vi "SPI Read Write.vi"(0 "SPI_Port":i8, 1 "SPI_CPOL":bool, 2 "SPI_CPHA":bool, 5 "SPI_Clock Divider":u32=20, 7 "SPI_Total Bytes":u16=1, 9 "SPI_Total Bits":u16=8, 11 "SPI_Write Data":u8[](array[numeric])=[0, 0], 12 "SPI_CS Active State":bool caption="SPI_CS\nActive State", 13 "SPI_CS":u8=1 format="%08b") -> (4 "SPI_Read Data":u8[](array[numeric]))   [LabVIEW 2019]
uses:
  Controls/FPGA SPI_FPGA SPI State.ctl
  <vilib>/rvi/Emulation/niFpgaSctlEmulationGetInTimedLoop.vi
  FPGA SPI_Globals.vi
  <vilib>/rvi/Emulation/niFpgaProcessEmulError.vi
  <vilib>/rvi/Emulation/niFpgaGetClockAttributes.vi
  <vilib>/rvi/Emulation/niFpgaEmulationReportErrorSimple.vi
  <vilib>/rvi/Emulation/niFpgaCriticalErrorInLSC.vi
  <vilib>/rvi/Emulation/niFpgaEmulationIsFPGAContextNoSignature.vi
  <vilib>/rvi/errors/niFpgaSetErrorForExecOnDevCompSimple.vi
  <vilib>/rvi/eio/common/nirviEmuReportErrorAndStop.vi
  <vilib>/rvi/DataTransferAndStorage/Container/Common/niFpgaContainerGetUniqueNameForEmu.vi
  <vilib>/rvi/FIFO/Fifo_Resource/nirvififoEmulationSetSize.vi
  <vilib>/rvi/FIFO/Fifo_Resource/nirviFifoEmulationQueueMgr.vi
  <instcachedir>/0/nirviFifoEmulationQueueMgr_E5CAEC123FF24DC58D834DCA3CDAA9B5.lvgen/nirviFifoEmulationQueueMgr_E5CAEC123FF24DC58D834DCA3CDAA9B5_002.vi
  <vilib>/rvi/FIFO/Fifo_Resource/nirvififoEmulationDetermineInputValidOut.vi
  <vilib>/rvi/FIFO/Fifo_Resource/nirvififoEmulationCreateLock.vi
  <vilib>/rvi/FIFO/Fifo_Resource/nirvififoEmulationObtainLock.vi
  <vilib>/rvi/FIFO/Fifo_Resource/nirvififoEmulationReleaseLock.vi
  <vilib>/rvi/occurrence/nirviWaitOnOccurrenceBase.vi
  <vilib>/rvi/errors/nirviReportUnexpectedCaseInternalError.vi
  <vilib>/rvi/errors/nirviReportUnexpectedCaseInternalError (U32).vi
  <vilib>/Utility/error.llb/Clear Errors.vi
  <vilib>/rvi/DataTransferAndStorage/Container/XNode/niFpgaContainer.xnode
  <vilib>/rvi/FIFO/Fifo_Resource/nirvififoEmulationWrite.vi
  <vilib>/rvi/FIFO/Fifo_Resource/nirvififoEmulationRead.vi
panel:
  out "SPI_Read Flag":bool
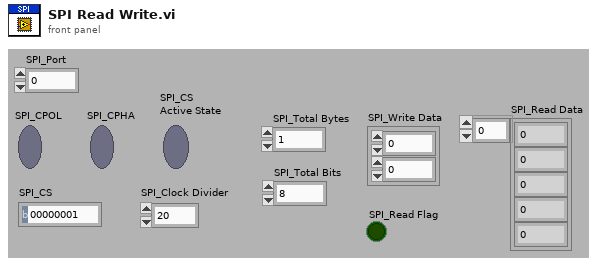
[diagram p1: front panel]
types:
  T1 = typedef "FPGA SPI_FPGA SPI State.ctl" = enum8{"Idle", "Read/Write SPI", "Configure"}
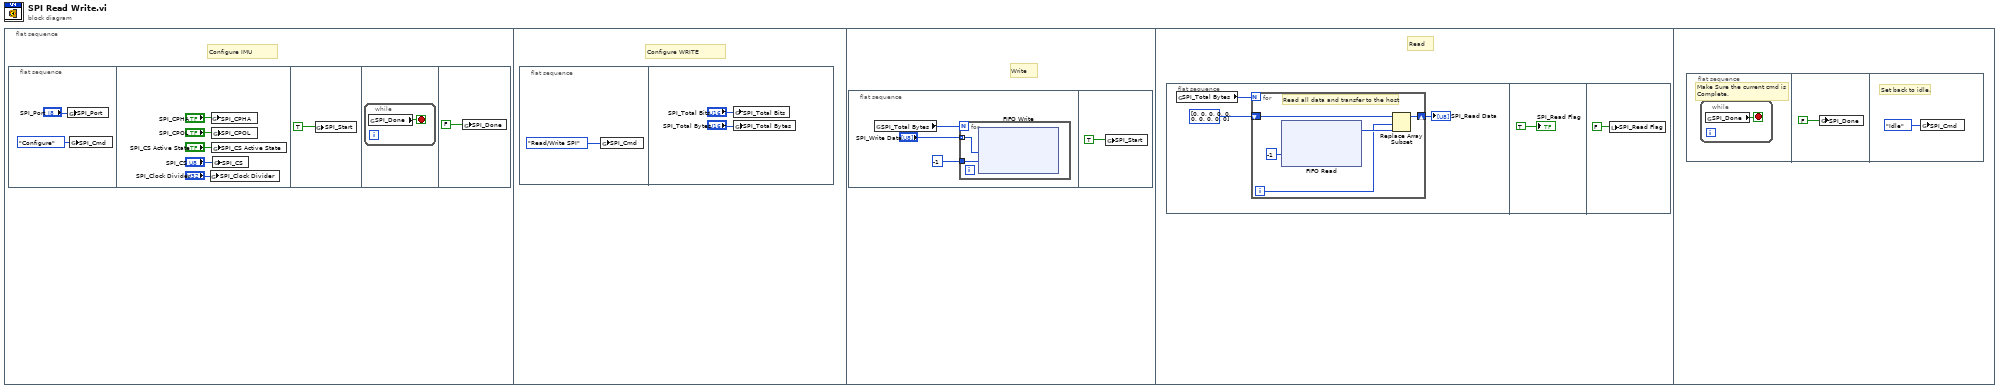
[diagram p0: block diagram]
diagram:
  n1 = flat-sequence {
    frame #0 {
      # "Configure IMU"
      n2 = flat-sequence {
        frame #0 {
          n3 = global write "FPGA SPI_Globals.vi" "SPI_Port"("SPI_Port") -> ()
          n4 = global write "FPGA SPI_Globals.vi" "SPI_Cmd"(FPGA_SPI_FPGA_SPI_State."Configure" ("SPI_Cmd")) -> ()
        }
        frame #1 {
          n5 = global write "FPGA SPI_Globals.vi" "SPI_Clock Divider"("SPI_Clock Divider") -> ()
          n6 = global write "FPGA SPI_Globals.vi" "SPI_CPHA"("SPI_CPHA") -> ()
          n7 = global write "FPGA SPI_Globals.vi" "SPI_CPOL"("SPI_CPOL") -> ()
          n8 = global write "FPGA SPI_Globals.vi" "SPI_CS Active State"("SPI_CS Active State") -> ()
          n9 = global write "FPGA SPI_Globals.vi" "SPI_CS"("SPI_CS") -> ()
        }
        frame #2 {
          n10 = global write "FPGA SPI_Globals.vi" "SPI_Start"(TRUE ("Write Flag")) -> ()
        }
        frame #3 {
          n11 = while {
            stop <- w9 stop-if-true
            n12 = global read "FPGA SPI_Globals.vi" "SPI_Done"() -> (w9:bool)
          }
        }
        frame #4 {
          n13 = global write "FPGA SPI_Globals.vi" "SPI_Done"(FALSE ("Done")) -> ()
        }
      }
    }
    frame #1 {
      # "Configure WRITE"
      n14 = flat-sequence {
        frame #0 {
          n15 = global write "FPGA SPI_Globals.vi" "SPI_Cmd"(FPGA_SPI_FPGA_SPI_State."Read/Write SPI" ("SPI_Cmd")) -> ()
        }
        frame #1 {
          n16 = global write "FPGA SPI_Globals.vi" "SPI_Total Bits"("SPI_Total Bits") -> ()
          n17 = global write "FPGA SPI_Globals.vi" "SPI_Total Bytes"("SPI_Total Bytes") -> ()
        }
      }
    }
    frame #2 {
      # "Write"
      n18 = flat-sequence {
        frame #0 {
          n19 = global read "FPGA SPI_Globals.vi" "SPI_Total Bytes"() -> (w14:u16)
          n20 = for {
            N: w14 -> [_]
            tunnel: -1 ("Timeout") -> [w18]
            tunnel: "SPI_Write Data" -> [w17] mode=indexing
            n21 = xnode ("FIFO Write")("Element"=w17, "Timeout"=w18) -> ()  [unwired: 1 in, 2 out]
          }
        }
        frame #1 {
          n22 = global write "FPGA SPI_Globals.vi" "SPI_Start"(TRUE ("Write Flag")) -> ()
        }
      }
    }
    frame #3 {
      # "Read"
      n23 = flat-sequence {
        frame #0 {
          n24 = global read "FPGA SPI_Globals.vi" "SPI_Total Bytes"() -> (w22:u16)
          n25 = for {
            N: w22 -> [_]
            shift-right: [w25] -> w21
            shift-left: u8[] [0, 0, 0, 0, 0, 0, 0, 0, 0, 0] ("array") -> [w23]
            i -> [w24]
            # "Read all data and transfer to the host"
            n26 = xnode ("FIFO Read")("Timeout"=-1) -> ("Element"=w27:u8)  [unwired: 1 in, 2 out]
            n27 = Replace Array Subset(array=w23, new element=w27, index=w24) -> (w25:u8[])
          }
          "SPI_Read Data" <- w21
        }
        frame #1 {
          "SPI_Read Flag" <- TRUE ("Read Flag")
        }
        frame #2 {
          n28 = local write "SPI_Read Flag"(FALSE ("Read Flag")) -> ()
        }
      }
    }
    frame #4 {
      n29 = flat-sequence {
        frame #0 {
          # "Make Sure the current cmd is\nComplete."
          n30 = while {
            stop <- w30 stop-if-true
            n31 = global read "FPGA SPI_Globals.vi" "SPI_Done"() -> (w30:bool)
          }
        }
        frame #1 {
          n32 = global write "FPGA SPI_Globals.vi" "SPI_Done"(FALSE ("Done")) -> ()
        }
        frame #2 {
          # "Set back to idle."
          n33 = global write "FPGA SPI_Globals.vi" "SPI_Cmd"(FPGA_SPI_FPGA_SPI_State."Idle" ("Type")) -> ()
        }
      }
    }
  }
